vi "Scaling data (recall mode).vi"(1 "Offset down":sgl format="%.2f", 2 "Offset up":sgl format="%.2f", 3 "Input data":sgl[](array[numeric]) format="%.2f") -> (0 "Scaled data":sgl[](array[numeric]) format="%.2f")   [LabVIEW 2010]
doc: "This VI scales the data from any range (also negative) into linear range in such a way that minimum input = 0.05 and maximum input = 0.95."
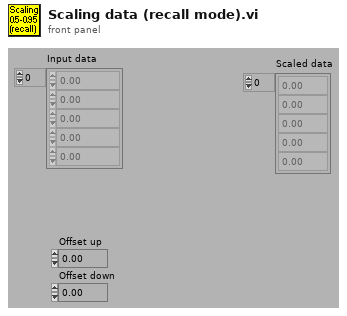
[diagram p1: front panel]
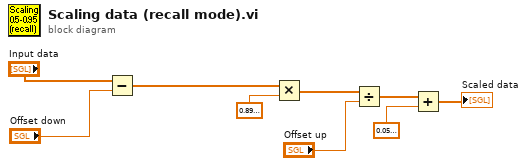
[diagram p0: block diagram]
diagram:
  n1 = Subtract(x="Input data", y="Offset down") -> (x-y=w3:sgl[])
  n2 = Multiply(x=w3, y=sgl 0.9 ("x")) -> (x*y=w8:sgl[])
  n3 = Divide(x=w8, y="Offset up") -> (x/y=w7:sgl[])
  n4 = Add(x=w7, y=sgl 0.05) -> (x+y=→"Scaled data":sgl[])
